vi "oa_Get CIC Decimation Filter Coefficients (Obsolete).vi"(7 "reset? (True)":bool=TRUE, 8 "alias protect in final transition":bool, 9 "stop band attenuation":u16(ring) items=["72 dB", "96 dB", "120 dB"], 11 "decimation/interpolation factor":i32=16) -> (0 "delay":i32, 1 "lp filter settings":T1={"coefficients"=[], "factor"=1} {"coefficients" format="%.2f"}, 2 "compensation filter settings":T1={"coefficients"=[], "factor"=1} {"coefficients" format="%.2f"}, 3 "CIC Settings":cluster{"Numeric":i32, i32, i32}, 4 "interpolation factor":i32)   [LabVIEW 2017]
uses:
  <vilib>/addons/_NISVFA/_Shared subVIs/Controls/OAT Decimation Filter.ctl
  <vilib>/addons/Sound and Vibration/Order Analysis/Resample Order Tracking/SoundVib_Resampling.lvlib
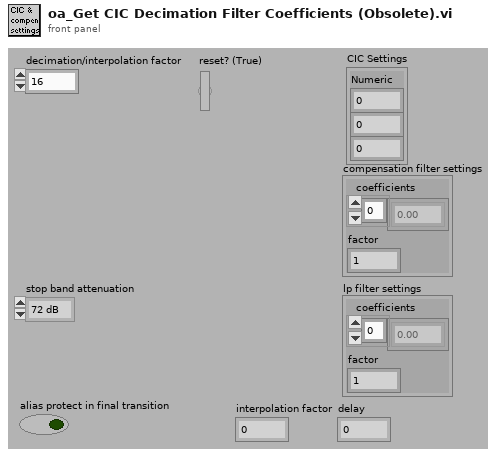
[diagram p1: front panel]
types:
  T1 = typedef "OAT Decimation Filter.ctl" = cluster{"coefficients":dbl[], "factor":i32}
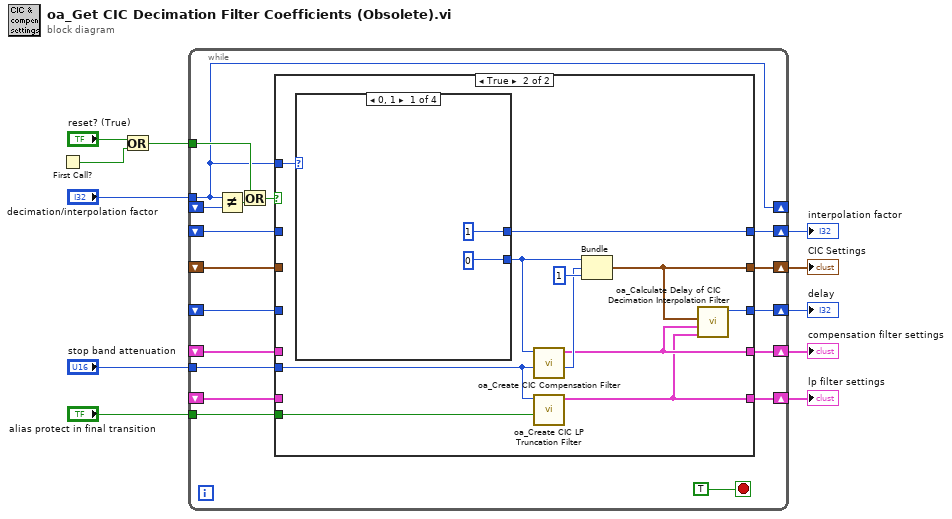
[diagram p0: block diagram]
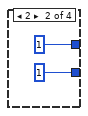
[diagram p3: hidden frame]
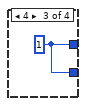
[diagram p4: hidden frame]
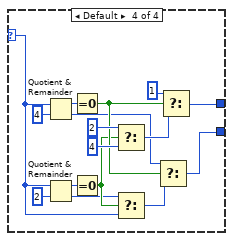
[diagram p5: hidden frame]
diagram:
  n1 = First Call?() -> (First Call?: T/F=w11:bool)
  n2 = Or(x="reset? (True)", y=w11) -> (x .or. y?=w9:bool)
  n3 = while {
    tunnel: w9 -> [w27]
    shift-right: [w14] -> _
    shift-left: _ -> [w29]
    tunnel: "decimation/interpolation factor" -> [w14]
    shift-right: [w24] -> w6
    shift-left: _ -> [w22]
    shift-right: [w23] -> w5
    shift-left: _ -> [w21]
    shift-right: [w20] -> w7
    shift-left: _ -> [w19]
    shift-right: [w18] -> w4
    shift-left: _ -> [w17]
    tunnel: "stop band attenuation" -> [w16]
    tunnel: "alias protect in final transition" -> [w15]
    shift-right: [w13] -> w1
    shift-left: _ -> [w12]
    stop <- TRUE stop-if-true
    n4 = Not Equal?(x=w14, y=w29) -> (x != y?=w28:bool)
    n5 = Or(x=w27, y=w28) -> (x .or. y?=w26:bool)
    n6 = case shown="True" w26 {
      tunnel: w14 -> [_ w45]
      tunnel: [w34 w37] -> w24
      tunnel: [w33 w36] -> w23
      tunnel: w22 -> [w34 _]
      tunnel: w21 -> [w33 _]
      tunnel: [w32 w38] -> w20
      tunnel: w19 -> [w32 _]
      tunnel: [w31 w43] -> w18
      tunnel: w17 -> [w31 _]
      tunnel: w16 -> [_ w40]
      tunnel: w15 -> [_ w39]
      tunnel: [w30 w35] -> w13
      tunnel: w12 -> [w30 _]
      frame False {
      }
      frame True {
        n7 = case shown="0, 1" w45 {
          selector: w45 -> [_ _ _ w51]
          tunnel: [1 1 w50 w62] -> w43
          tunnel: [0 1 w50 w52] -> w41
          frame 0, 1 {
          }
          frame 2 {
          }
          frame 4 {
            w50 = 1
          }
          frame Default {
            n8 = Quotient & Remainder(x=w51, y=4) -> (x-y*floor(x/y)=w65:i32, floor(x/y)=w54:i32)
            n9 = Quotient & Remainder(x=w51, y=2) -> (x-y*floor(x/y)=w64:i32, floor(x/y)=w53:i32)
            n10 = Equal To 0?(x=w65) -> (x = 0?=w57:bool)
            n11 = Equal To 0?(x=w64) -> (x = 0?=w55:bool)
            n12 = Select(t=2, s=w55, f=4) -> (s? t:f=w58:i32)
            n13 = Select(t=w53, s=w55, f=w51) -> (s? t:f=w56:i32)
            n14 = Select(t=w54, s=w57, f=w56) -> (s? t:f=w52:i32)
            n15 = Select(t=1, s=w57, f=w58) -> (s? t:f=w62:i32)
          }
        }
        n16 = call <vilib>:"oa_Create CIC Compensation Filter.vi"("stop band attenuation"=w40, "decimation factor"=w41) -> ("stage"=w42:i32, "compensation filter settings"=w37:T1)  [unwired: 8 in]
        n17 = call <vilib>:"oa_Create CIC LP Truncation Filter.vi"("alias protect in final transition"=w39, "stop band attenuation"=w40) -> ("lp filter settings"=w36:T1)  [unwired: 9 in]
        n18 = Bundle("Numeric"=w41, "stage"=w42, 1) -> (w38:cluster{"Numeric":i32, "stage":i32, i32})  [unwired: 1 in]
        n19 = call <vilib>:"oa_Calculate Delay of CIC Decimation Interpolation Filter.vi"("lp filter settings"=w36, "compensation filter settings"=w37, "CIC decimation setting"=w38) -> ("delay"=w35:i32)  [unwired: 8 in]
      }
    }
  }
  "CIC Settings" <- w7
  "compensation filter settings" <- w6
  "lp filter settings" <- w5
  "interpolation factor" <- w4
  "delay" <- w1
